vi "q2 horse running while loop.vi"() -> ()   [LabVIEW 2018]
panel:
  out "Ring 2":u16(ring)
  in  "n (for)":dbl
  in  "stop":bool
  in  "n (while)":dbl
  out "Ring":u16(ring)
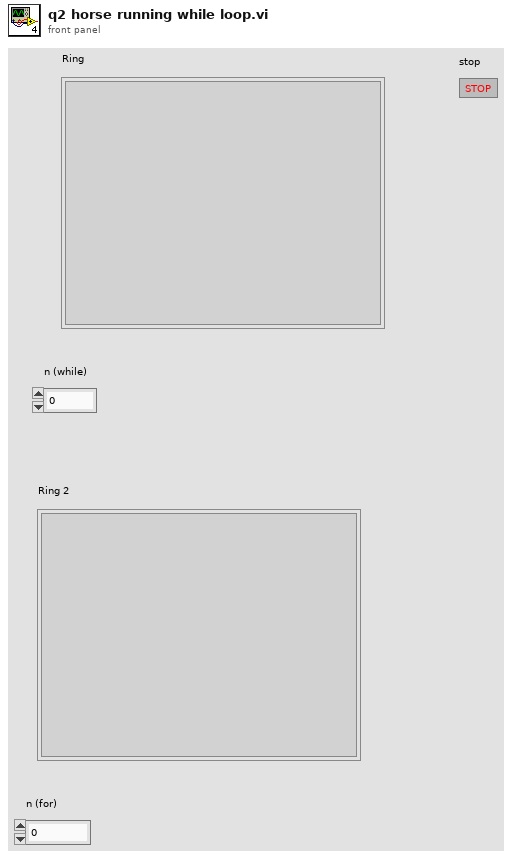
[diagram p1: front panel]
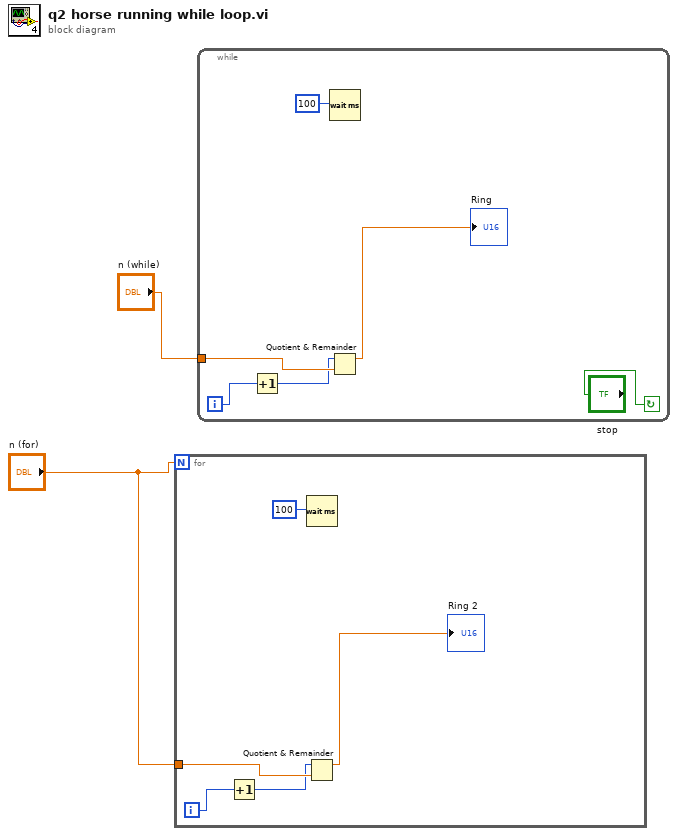
[diagram p0: block diagram]
diagram:
  n1 = for {
    N: "n (for)" -> [_]
    tunnel: "n (for)" -> [w4]
    i -> [w7]
    n2 = Increment(x=w7) -> (x+1=w3:i32)
    n3 = Wait (ms)(milliseconds to wait=100) -> ()  [unwired: 1 out]
    n4 = Quotient & Remainder(x=w3, y=w4) -> (x-y*floor(x/y)=→"Ring 2":dbl)  [unwired: 1 out]
  }
  n5 = while {
    tunnel: "n (while)" -> [w9]
    i -> [w12]
    stop <- "stop" continue-if-true
    n6 = Increment(x=w12) -> (x+1=w8:i32)
    n7 = Wait (ms)(milliseconds to wait=100) -> ()  [unwired: 1 out]
    n8 = Quotient & Remainder(x=w8, y=w9) -> (x-y*floor(x/y)=→"Ring":dbl)  [unwired: 1 out]
  }
